vi "Compile - Buffered Channel Refs.vi"(6 "Packet Name":string, 7 "Timestamp Present?":bool, 8 "error in (no error)":errorcluster, 11 "Item Ref in":T1 format="%.0x") -> (0 "error out":errorcluster, 3 "Item Ref out":T1 format="%.0x", 4 "Tx Ref Array":T2(array[cluster]) {"VS Refs" format="%.0x"})   [LabVIEW 2016, in "UDP-Custom-Device System Explorer.lvlib"]
uses:
  UDP-Custom-Device System Explorer.lvlib
  <vilib>/NI Veristand/Custom Device API/Custom Device Item Ref.ctl
  Property Accessors/Tx Packet Accessors.lvlib
  <vilib>/NI VeriStand/Custom Device API/Custom Device API.lvlib
  Property Accessors/Buffered Data Packet.lvlib
  <vilib>/NI VeriStand/Custom Device Tools/Custom Device Utility Library/Custom Device Utility Library.lvlib
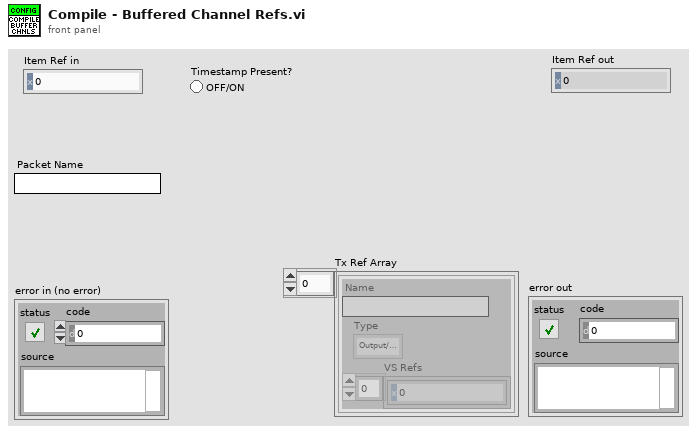
[diagram p1: front panel]
types:
  T1 = typedef "Custom Device API.lvlib/Custom Device Item Ref.ctl" = u64
  T2 = cluster{"Name":string, "Type":enum16{"Output/Write", "Input/Read", "Input/ReadWrite"}, "VS Refs":T1[]}[]
  T3 = enum16{"Output/Write", "Input/Read", "Input/ReadWrite"}
  T4 = cluster{"Name":string, "Type":enum16{"Output/Write", "Input/Read", "Input/ReadWrite"}, "VS Refs":T1[]}
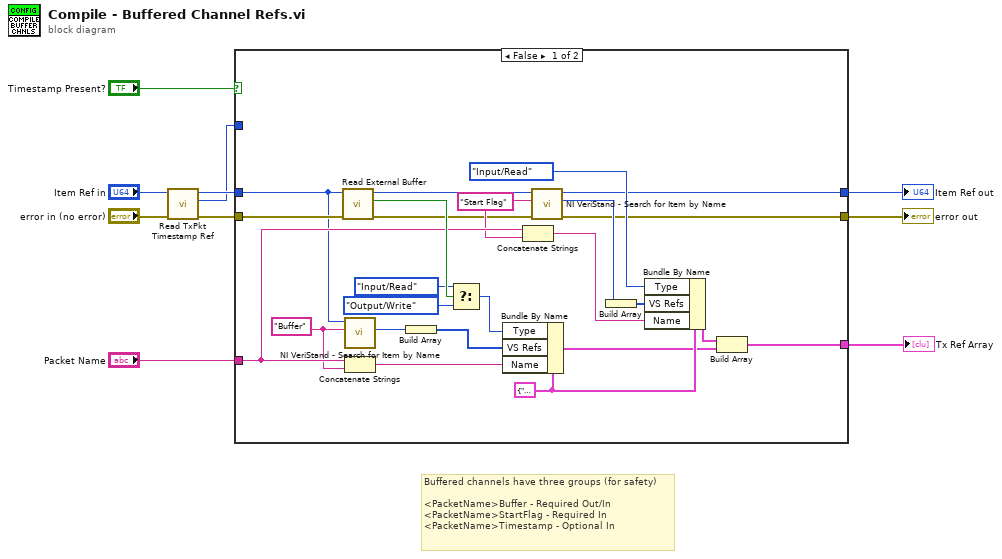
[diagram p0: block diagram]
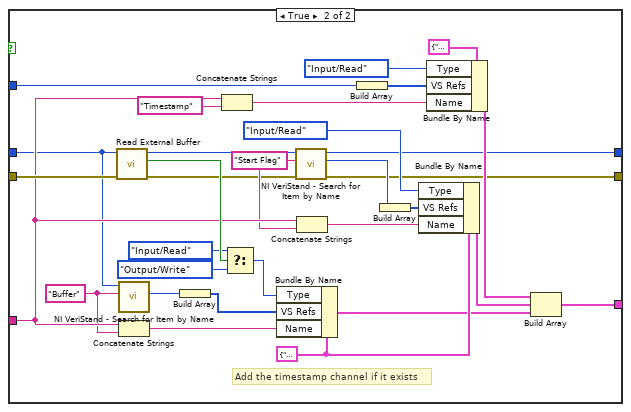
[diagram p2: hidden frame]
diagram:
  # "Buffered channels have three groups (for safety)\n\n<PacketName>Buffer - Required Out/In\n<PacketName>StartFlag - Required In\n<PacketName>Timestamp - Optional In"
  n1 = call "Read TxPkt Timestamp Ref.vi"("error in (no error)"="error in (no error)", "Node Ptr"="Item Ref in") -> ("error out"=w9:errorcluster, "Timestamp Ref"=w8:T1, "Node Ptr out"=w10:T1)  [unwired: 7 in]
  n2 = case shown="False" "Timestamp Present?" {
    tunnel: [w14 w38] -> w2
    tunnel: "Packet Name" -> [w25 w50]
    tunnel: [w20 w52] -> w1
    tunnel: w10 -> [w13 w37]
    tunnel: w9 -> [w34 w65]
    tunnel: w8 -> [_ w47]
    tunnel: [w16 w40] -> w3
    frame False {
      w18 = "Start Flag" ("Item GUID")
      w12 = "Buffer" ("Item GUID")
      w23 = T4 {"Name"="", "Type"=enum."Output/Write", "VS Refs"=[]} ("Group")
      n3 = call "Read External Buffer.vi"("error in (no error)"=w34, "Node Ptr"=w13) -> ("error out"=w17:errorcluster, "External Buffer"=w31:bool, "Node Ptr out"=w19:T1)  [unwired: 7 in]
      n4 = call <vilib>:"NI VeriStand - Search for Item by Name.vi"("Item Name"=w12, "Section Ref in"=w13) -> ("Item Ref"=w11:T1)  [unwired: 6 in, 3 out]
      n5 = Concatenate Strings(w25, w12) -> (w33:string)
      n6 = Build Array(w11) -> (w32:T1[])
      n7 = Select(t=T3."Input/Read" ("Type"), s=w31, f=T3."Output/Write" ("Type")) -> (s? t:f=w28:T3)
      n8 = Bundle By Name(cluster=w23, "Type"=w28, "VS Refs"=w32, "Name"=w33) -> (w21:T4)
      n9 = Concatenate Strings(w25, w18) -> (w24:string)
      n10 = call <vilib>:"NI VeriStand - Search for Item by Name.vi"("error in"=w17, "Item Name"=w18, "Section Ref in"=w19) -> ("error out"=w14:errorcluster, "Item Ref"=w15:T1, "Section Ref out"=w16:T1)  [unwired: 5 in, 1 out]
      n11 = Build Array(w15) -> (w26:T1[])
      n12 = Bundle By Name(cluster=w23, "Type"=T3."Input/Read", "VS Refs"=w26, "Name"=w24) -> (w22:T4)
      n13 = Build Array(w22, w21) -> (w20:T2)
    }
    frame True {
      w42 = "Start Flag" ("Item GUID")
      w36 = "Buffer" ("Item GUID")
      w55 = T4 {"Name"="", "Type"=enum."Output/Write", "VS Refs"=[]} ("Group")
      # "Add the timestamp channel if it exists"
      n14 = call "Read External Buffer.vi"("error in (no error)"=w65, "Node Ptr"=w37) -> ("error out"=w41:errorcluster, "External Buffer"=w62:bool, "Node Ptr out"=w43:T1)  [unwired: 7 in]
      n15 = call <vilib>:"NI VeriStand - Search for Item by Name.vi"("Item Name"=w36, "Section Ref in"=w37) -> ("Item Ref"=w35:T1)  [unwired: 6 in, 3 out]
      n16 = Concatenate Strings(w50, w36) -> (w64:string)
      n17 = Build Array(w35) -> (w63:T1[])
      n18 = Concatenate Strings(w50, "Timestamp" ("Item GUID")) -> (w48:string)
      n19 = Select(t=T3."Input/Read" ("Type"), s=w62, f=T3."Output/Write" ("Type")) -> (s? t:f=w59:T3)
      n20 = Bundle By Name(cluster=w55, "Type"=w59, "VS Refs"=w63, "Name"=w64) -> (w53:T4)
      n21 = call <vilib>:"NI VeriStand - Search for Item by Name.vi"("error in"=w41, "Item Name"=w42, "Section Ref in"=w43) -> ("error out"=w38:errorcluster, "Item Ref"=w39:T1, "Section Ref out"=w40:T1)  [unwired: 5 in, 1 out]
      n22 = Concatenate Strings(w50, w42) -> (w56:string)
      n23 = Build Array(w47) -> (w49:T1[])
      n24 = Build Array(w39) -> (w57:T1[])
      n25 = Bundle By Name(cluster=w55, "Type"=T3."Input/Read", "VS Refs"=w57, "Name"=w56) -> (w54:T4)
      n26 = Bundle By Name(cluster=T4 {"Name"="", "Type"=enum."Output/Write", "VS Refs"=[]} ("Group"), "Type"=T3."Input/Read", "VS Refs"=w49, "Name"=w48) -> (w44:T4)
      n27 = Build Array(w44, w54, w53) -> (w52:T2)
    }
  }
  "Tx Ref Array" <- w1
  "error out" <- w2
  "Item Ref out" <- w3
